vi "Write SPI Channel (0).vi"(8 "error in (no error)":errorcluster, 10 "SPI Channel (0)":u8, 11 "LINX SPI in":refnum<class "LINX SPI.lvclass">) -> (0 "error out":errorcluster, 3 "LINX SPI out":refnum<class "LINX SPI.lvclass">)   [LabVIEW 2020, in "LINX SPI.lvclass"]
uses:
  LINX SPI.lvclass
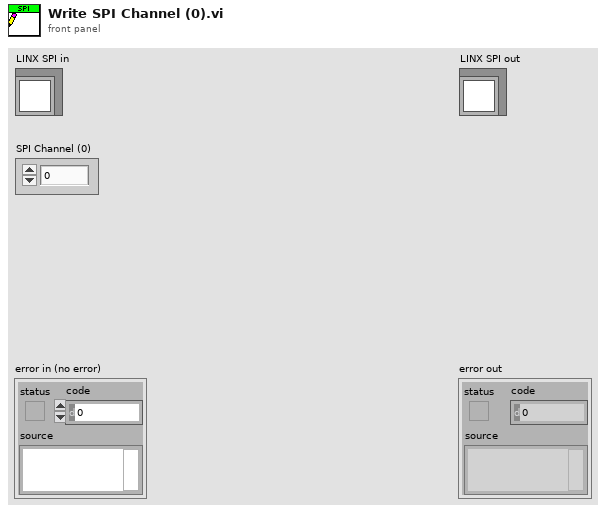
[diagram p1: front panel]
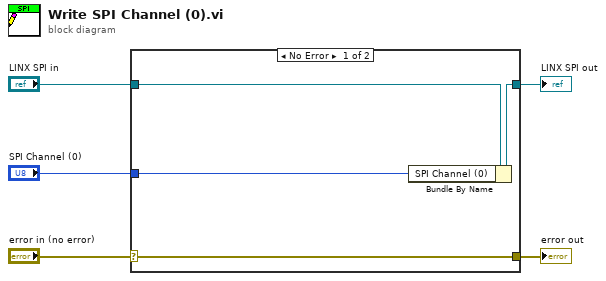
[diagram p0: block diagram]
diagram:
  n1 = case shown="No Error" "error in (no error)" {
    selector: "error in (no error)" -> [w9 w10]
    tunnel: [w9 w10] -> w4
    tunnel: [w7 w11] -> w2
    tunnel: "LINX SPI in" -> [w8 w11]
    tunnel: "SPI Channel (0)" -> [w6 _]
    frame No Error {
      n2 = Bundle By Name(cluster=w8, "SPI Channel (0)"=w6) -> (w7:refnum<class "LINX SPI.lvclass">)
    }
    frame Error {
    }
  }
  "error out" <- w4
  "LINX SPI out" <- w2
